vi "Init.vi"(8 "error in (no error)":errorcluster, 9 "Board (Default)":string, 10 "Resource (None)":refnum<class "DeployResource.lvclass">, 11 "Platform (None)":refnum<class "DeployPlatform.lvclass">) -> (0 "error out":errorcluster, 3 "Device out":refnum<class "Device.lvclass">)   [LabVIEW 2020, in "PicoG-Core.lvlib" / "Device.lvclass"]
uses:
  Device.lvclass
  DeployPlatform/DeployPlatform.lvclass
  DeployResource/DeployResource.lvclass
  Device.lvclass/Device.ctl
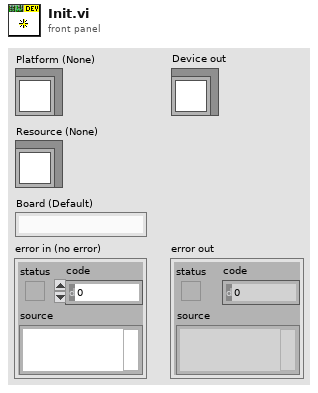
[diagram p1: front panel]
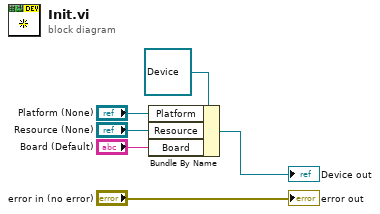
[diagram p0: block diagram]
diagram:
  n1 = Bundle By Name(cluster=refnum<class "Device.lvclass"> refnum ("Device in"), "Platform"="Platform (None)", "Resource"="Resource (None)", "Board"="Board (Default)") -> (→"Device out":refnum<class "Device.lvclass">)
  "error out" <- "error in (no error)"
